vi "Need_Interpolation.vi"(1 "Matrix with txt":string[][](array[string]), 2 "Number of Rows":i32) -> (0 "isNotFive?":bool)   [LabVIEW 2014]
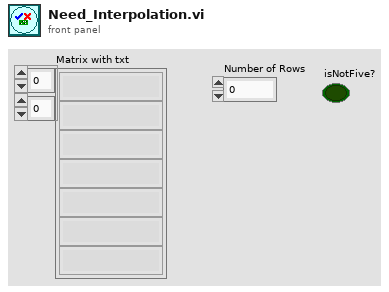
[diagram p1: front panel]
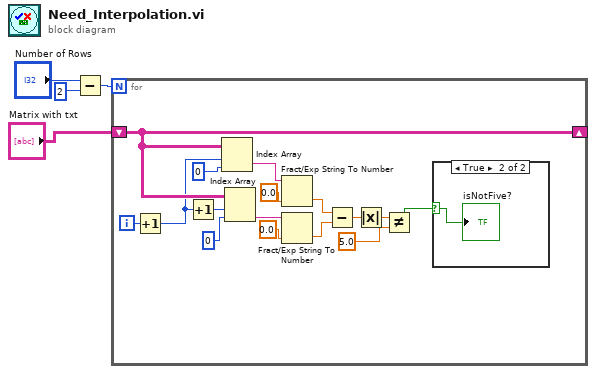
[diagram p0: block diagram]
diagram:
  n1 = Subtract(x="Number of Rows", y=2) -> (x-y=w1:i32)
  n2 = for {
    N: w1 -> [_]
    shift-right: [w10] -> _
    shift-left: "Matrix with txt" -> [w10]
    i -> [w9]
    n3 = Increment(x=w9) -> (x+1=w8:i32)
    n4 = Increment(x=w8) -> (x+1=w6:i32)
    n5 = Index Array(array=w10, index (row)=w8, index (col)=0 ("disabled index (col)")) -> (element=w7:string)
    n6 = Index Array(array=w10, index (row)=w6, index (col)=0 ("disabled index (col)")) -> (element=w11:string)
    n7 = Fract/Exp String To Number(string=w7, default (0 dbl)=0.0 ("default (0 DBL)")) -> (number=w16:dbl)  [unwired: 2 in, 1 out]
    n8 = Fract/Exp String To Number(string=w11, default (0 dbl)=0.0 ("default (0 DBL)")) -> (number=w15:dbl)  [unwired: 2 in, 1 out]
    n9 = Subtract(x=w16, y=w15) -> (x-y=w14:dbl)
    n10 = Absolute Value(x=w14) -> (abs(x)=w13:dbl)
    n11 = Not Equal?(x=w13, y=5.0) -> (x != y?=w5:bool)
    n12 = case shown="True" w5 {
      selector: w5 -> [_ w21]
      frame False {
      }
      frame True {
        "isNotFive?" <- w21
      }
    }
  }
